vi "Script_Timing_Extract_Wfms.vi"(7 "Script Text":string="script PireneaGas2sExcitAcq8s\n   wait until scriptTrigger0 \n   wait dd\n   generate AutLaserOn\n   wait 49000\n   generate AutLaserOnFilterOff\n   wait 1000\n   wait 600\n   generate AutLaserOnFilterOffTrapStart\n   wait 300\n   generate AutLaserOnFilterOffTrapStop\n   wait 2000\n   generate AutLaserOnFilterOn\n   wait 47100\n   generate AutLaserOff\n   wait 1950000\n   generate Gas1On\n   wait 150000\n   generate Gas1Off\n   wait 5850000\n   generate ExcitAcq\n   wait 1000000\n   generate FilterOff\n   wait 1000\n   generate FilterOffEmptyingStart\n   wait 1000000\n   generate FilterOffEmptyingStop\n   wait 2000\n   generate Zeros\nend script", 8 "error in (no error)":errorcluster, 9 "Script File":string="Adiabatic.txt", 10 "Script Path":path=path "D:/PIRENEA/SEQUENCE_SCRIPTS") -> (0 "error out":errorcluster, 2 "Script Checked":string, 3 "Table of Waveforms":string[](array[string]))   [LabVIEW 2017]
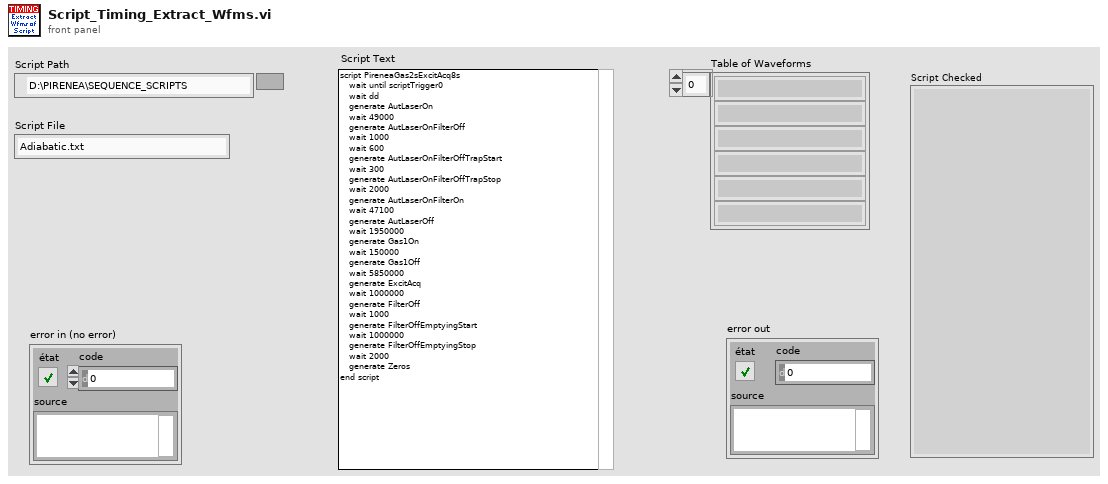
[diagram p1: front panel]
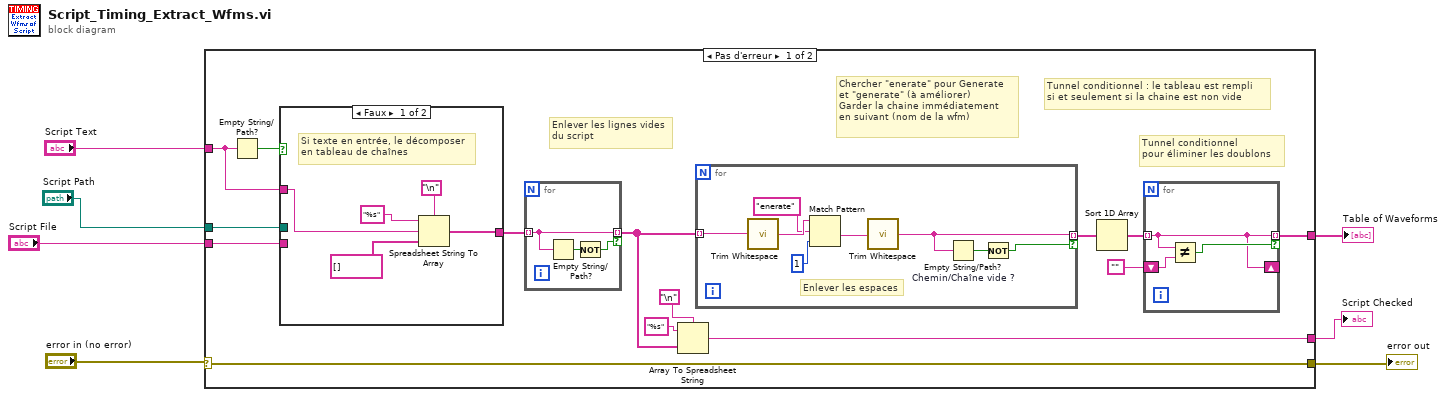
[diagram p0: block diagram]
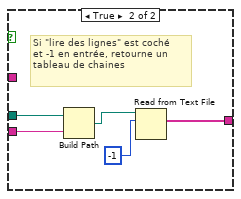
[diagram p2: hidden frame]
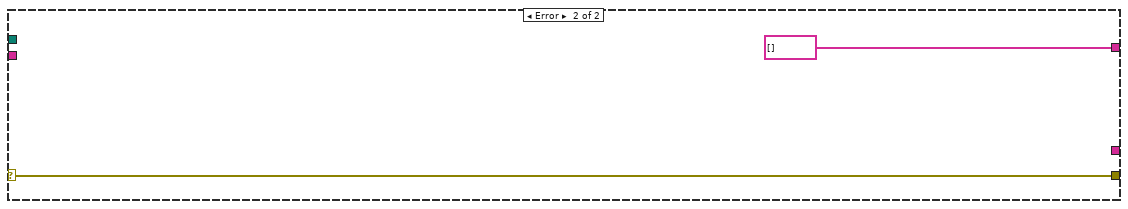
[diagram p3: hidden frame]
diagram:
  n1 = case shown="Pas d'erreur" "error in (no error)" {
    selector: "error in (no error)" -> [w19 w47]
    tunnel: "Script File" -> [w21 _]
    tunnel: [w19 w47] -> w5
    tunnel: "Script Path" -> [w20 _]
    tunnel: [w15 string[] []] -> w3
    tunnel: "Script Text" -> [w13 _]
    tunnel: [w8 _] -> w1
    frame No Error {
      # "Enlever les lignes vides\ndu script"
      # "Tunnel conditionnel\npour éliminer les doublons"
      # "Tunnel conditionnel : le tableau est rempli\nsi et seulement si la chaine est non vide"
      # "Chercher \"enerate\" pour Generate\net \"generate\" (à améliorer)\nGarder la chaine immédiatement\nen suivant (nom de la wfm)"
      n2 = Empty String/Path?(string/path=w13) -> (empty?=w14:bool)
      n3 = case shown="Faux" w14 {
        tunnel: w21 -> [_ w34]
        tunnel: w20 -> [_ w33]
        tunnel: [w25 w30] -> w12
        tunnel: w13 -> [w26 _]
        frame False {
          # "Si texte en entrée, le décomposer\nen tableau de chaînes"
          n4 = Spreadsheet String To Array(delimiter (Tab)="\n", format string="%s" ("chaîne de format"), spreadsheet string=w26, array type (2D Dbl)=string[] []) -> (array=w25:string[])
        }
        frame True {
          # "Si \"lire des lignes\" est coché\net -1 en entrée, retourne un tableau de chaines"
          n5 = Build Path(base path=w33, name or relative path=w34) -> (appended path=w32:path)
          n6 = Read from Text File(file (use dialog)=w32, count=-1 ("nombre")) -> (text=w30:string[])  [unwired: 2 in, 3 out]
        }
      }
      n7 = for {
        tunnel: w12 -> [w23] mode=indexing
        tunnel: [w23] -> w11 mode=indexing if=w22
        n8 = Empty String/Path?(string/path=w23) -> (empty?=w24:bool)
        n9 = Not(x=w24) -> (.not. x?=w22:bool)
      }
      n10 = Array To Spreadsheet String(delimiter (Tab)="\n", array=w11, 3:"%s" ("chaîne de format")) -> (spreadsheet string=w8:string)
      n11 = for {
        tunnel: w11 -> [w45] mode=indexing
        tunnel: [w38] -> w16 mode=indexing if=w39
        # "Enlever les espaces"
        n12 = call <vilib>:"Trim Whitespace.vi"("string"=w45) -> ("trimmed string"=w44:string)  [unwired: 1 in]
        n13 = Match Pattern(string=w44, regular expression="enerate" ("expression régulière"), offset (0)=1) -> (after substring=w41:string)  [unwired: 3 out]
        n14 = call <vilib>:"Trim Whitespace.vi"("string"=w41) -> ("trimmed string"=w38:string)  [unwired: 1 in]
        n15 = Empty String/Path? "Chemin/Chaîne vide ?"(string/path=w38) -> (empty?=w40:bool)
        n16 = Not(x=w40) -> (.not. x?=w39:bool)
      }
      n17 = Sort 1D Array(array=w16) -> (sorted array=w18:string[])
      n18 = for {
        tunnel: w18 -> [w35] mode=indexing
        shift-right: [w35] -> _
        shift-left: "" -> [w37]
        tunnel: [w35] -> w15 mode=indexing if=w36
        n19 = Not Equal?(x=w35, y=w37) -> (x != y?=w36:bool)
      }
    }
    frame Error {
    }
  }
  "error out" <- w5
  "Table of Waveforms" <- w3
  "Script Checked" <- w1
